vi "CropLiftPos.vi"(10 "Position":dbl) -> (2 "New Position":dbl)   [LabVIEW 2015]
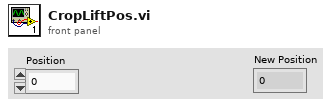
[diagram p1: front panel]
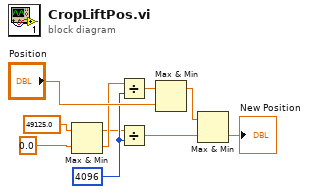
[diagram p0: block diagram]
diagram:
  w5 = 4096
  n1 = Max & Min(x=49125.0, y=0.0) -> (max(x,y)=w3:dbl, min(x,y)=w4:dbl)
  n2 = Divide(x=w4, y=w5) -> (x/y=w6:dbl)
  n3 = Divide(x=w3, y=w5) -> (x/y=w7:dbl)
  n4 = Max & Min(x=w6, y="Position") -> (max(x,y)=w9:dbl)  [unwired: 1 out]
  n5 = Max & Min(x=w9, y=w7) -> (min(x,y)=→"New Position":dbl)  [unwired: 1 out]
